vi "Set Item Configurations.vi"(8 "error in (no error)":errorcluster, 10 "Item Configurations":refnum<class "Item Configuration.lvclass">[](array[class]), 11 "Create Project Model in":refnum<class "Create Project Model.lvclass">) -> (0 "error out":errorcluster, 3 "Create Project Model out":refnum<class "Create Project Model.lvclass">)   [LabVIEW 2013, in "Create Project Model.lvlib" / "Create Project Model.lvclass"]
uses:
  Create Project Model.lvclass
  Common/Item Configuration/Item Configuration/Item Configuration.lvclass
  Create Project Model.lvclass/Create Project Model.ctl
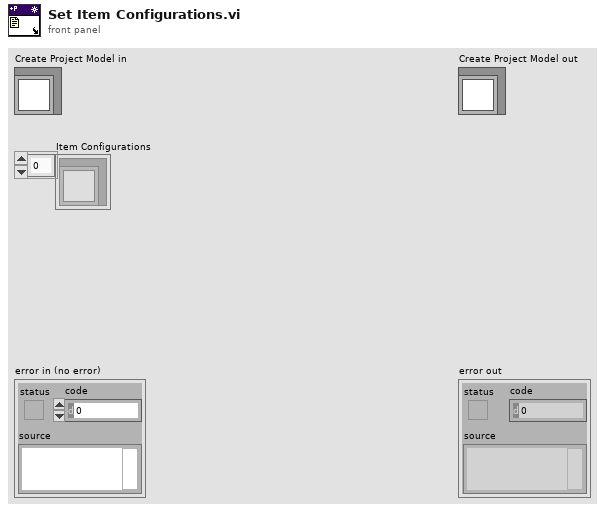
[diagram p1: front panel]
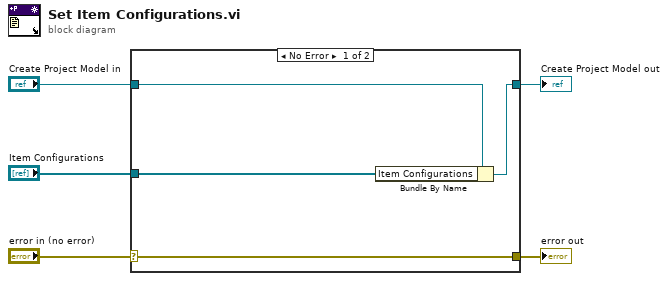
[diagram p0: block diagram]
diagram:
  n1 = case shown="No Error" "error in (no error)" {
    selector: "error in (no error)" -> [w9 w10]
    tunnel: [w9 w10] -> w4
    tunnel: [w7 w11] -> w2
    tunnel: "Create Project Model in" -> [w8 w11]
    tunnel: "Item Configurations" -> [w6 _]
    frame No Error {
      n2 = Bundle By Name(cluster=w8, "Item Configurations"=w6) -> (w7:refnum<class "Create Project Model.lvclass">)
    }
    frame Error {
    }
  }
  "error out" <- w4
  "Create Project Model out" <- w2
